vi "Write Actor Queues.vi"(10 "Base Actor Queues":T1, 11 "Template in":refnum<class "Template.lvclass">) -> (3 "Template out":refnum<class "Template.lvclass">)   [LabVIEW 2020, in "Template.lvlib" / "Template.lvclass"]
doc: "Sets the actor queues"
uses:
  Template.lvclass
  typedefs/base actor queues.ctl
  Template.lvclass/Template.ctl
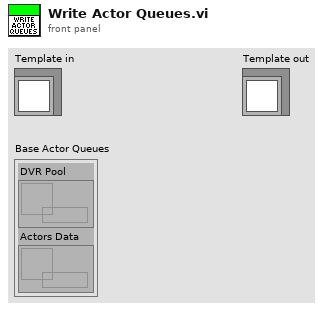
[diagram p1: front panel]
types:
  T1 = typedef "Template.lvlib/Template.lvclass/base actor queues.ctl" = cluster{"DVR Pool":refnum<queue>, "Actors Data":refnum<queue>}
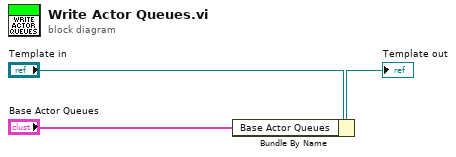
[diagram p0: block diagram]
diagram:
  n1 = Bundle By Name(cluster="Template in", "Base Actor Queues"="Base Actor Queues") -> (→"Template out":refnum<class "Template.lvclass">)
